vi "Untitled 1 (SubVI).vi"(9 "Right Encoder":i32, 10 "Left Encoder":i32, 11 "PostionTarget(Counts)":i32) -> (2 "Boolean 2":bool, 3 "Boolean":bool)   [LabVIEW 2017, in "Autonomous.lvlib"]
uses:
  Autonomous.lvlib
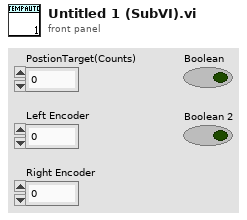
[diagram p1: front panel]
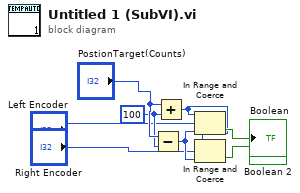
[diagram p0: block diagram]
diagram:
  w3 = 100 ("y")
  n1 = Subtract(x="PostionTarget(Counts)", y=w3) -> (x-y=w6:i32)
  n2 = Add(x="PostionTarget(Counts)", y=w3) -> (x+y=w5:i32)
  n3 = In Range and Coerce(upper limit=w5, x="Left Encoder", lower limit=w6) -> (In Range?=→"Boolean":bool)  [unwired: 1 out]
  n4 = In Range and Coerce(upper limit=w5, x="Right Encoder", lower limit=w6) -> (In Range?=→"Boolean 2":bool)  [unwired: 1 out]
